vi "09_Notifier_vs_Fronta.vi"() -> ()   [LabVIEW 2019]
panel:
  out "Fronta":dbl(graph)
  out "Notifier":dbl(graph)
  in  "Boolean":bool
  in  "stop":bool
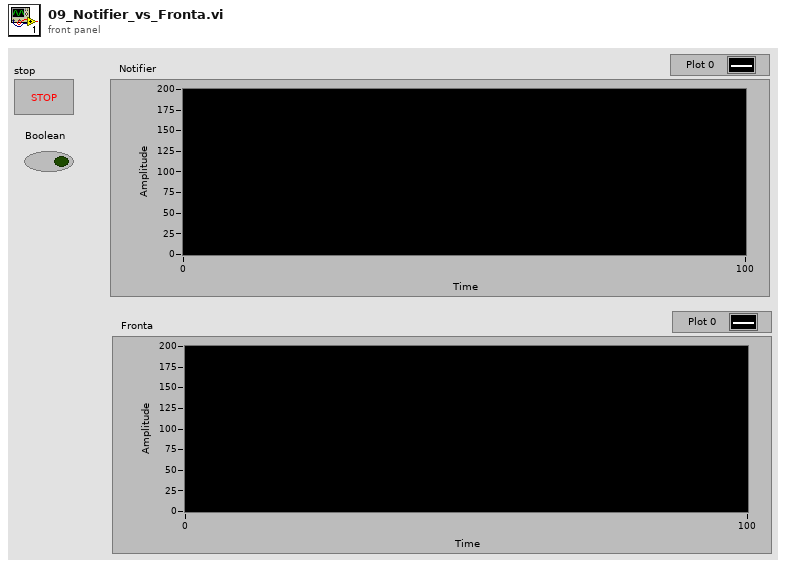
[diagram p1: front panel]
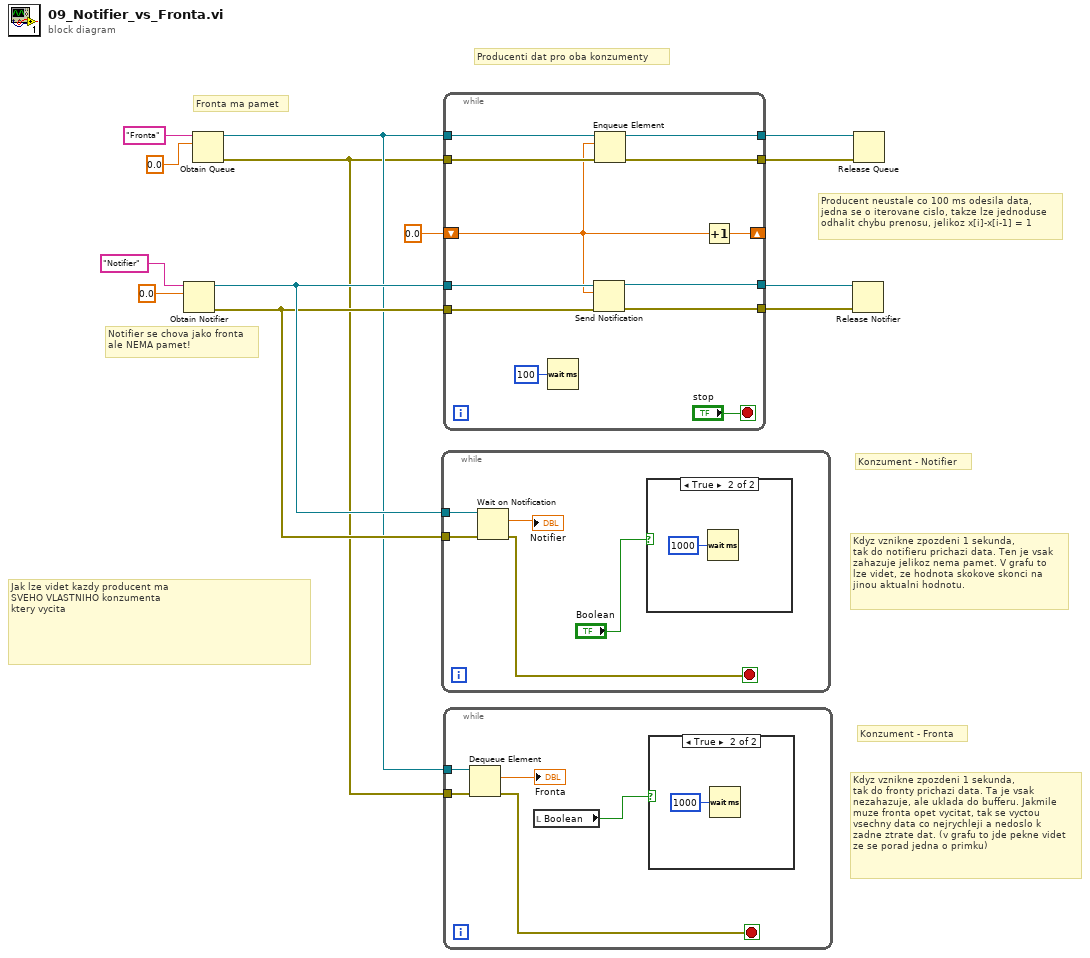
[diagram p0: block diagram]
diagram:
  # "Jak lze videt kazdy producent ma\nSVEHO VLASTNIHO konzumenta\nktery vycita"
  # "Konzument - Fronta"
  # "Konzument - Notifier"
  # "Producenti dat pro oba konzumenty"
  # "Kdyz vznikne zpozdeni 1 sekunda,\ntak do fronty prichazi data. Ta je vsak\nnezahazuje, ale uklada do bufferu. Jakmile\nmuze fronta opet vycitat, tak se vyctou \nvsechny data co nejrychleji a nedoslo k\nzadne ztrate dat. (v grafu to jde pekne videt\nze se porad jedna o primku)"
  # "Producent neustale co 100 ms odesila data,\njedna se o iterovane cislo, takze lze jednoduse\nodhalit chybu prenosu, jelikoz x[i]-x[i-1] = 1"
  # "Kdyz vznikne zpozdeni 1 sekunda,\ntak do notifieru prichazi data. Ten je vsak\nzahazuje jelikoz nema pamet. V grafu to \nlze videt, ze hodnota skokove skonci na \njinou aktualni hodnotu."
  # "Notifier se chova jako fronta\nale NEMA pamet!"
  # "Fronta ma pamet"
  n1 = Obtain Notifier(name (unnamed)="Notifier", notification data type=0.0) -> (notifier out=w8:refnum<notifier>, error out=w7:errorcluster)  [unwired: 2 in, 1 out]
  n2 = Obtain Queue(name (unnamed)="Fronta", element data type=0.0) -> (queue out=w2:refnum<queue>, error out=w1:errorcluster)  [unwired: 3 in, 1 out]
  n3 = while {
    tunnel: w8 -> [w17]
    tunnel: w7 -> [w18]
    stop <- w16 stop-if-true
    n4 = Wait on Notification(notifier=w17, error in (no error)=w18) -> (notification=→"Notifier":dbl, error out=w16:errorcluster)  [unwired: 2 in, 2 out]
    n5 = case shown="True" "Boolean" {
      frame False {
      }
      frame True {
        n6 = Wait (ms)(milliseconds to wait=u32 1000) -> ()  [unwired: 1 out]
      }
    }
  }
  n7 = while {
    tunnel: w8 -> [w31]
    tunnel: w7 -> [w30]
    shift-right: [w28] -> _
    shift-left: 0.0 -> [w20]
    tunnel: [w27] -> w10
    tunnel: [w26] -> w9
    tunnel: w2 -> [w24]
    tunnel: w1 -> [w23]
    tunnel: [w22] -> w4
    tunnel: [w21] -> w3
    stop <- "stop" stop-if-true
    n8 = Wait (ms)(milliseconds to wait=u32 100) -> ()  [unwired: 1 out]
    n9 = Send Notification(notification=w20, notifier=w31, error in (no error)=w30) -> (notifier out=w27:refnum<notifier>, error out=w26:errorcluster)
    n10 = Enqueue Element(queue=w24, element=w20, error in (no error)=w23) -> (queue out=w22:refnum<queue>, error out=w21:errorcluster)  [unwired: 1 in, 1 out]
    n11 = Increment(x=w20) -> (x+1=w28:dbl)
  }
  n12 = while {
    tunnel: w2 -> [w35]
    tunnel: w1 -> [w34]
    stop <- w32 stop-if-true
    n13 = Dequeue Element(queue=w35, error in (no error)=w34) -> (element=→"Fronta":dbl, error out=w32:errorcluster)  [unwired: 1 in, 2 out]
    n14 = local read "Boolean"() -> (w36:bool)
    n15 = case shown="True" w36 {
      frame False {
      }
      frame True {
        n16 = Wait (ms)(milliseconds to wait=u32 1000) -> ()  [unwired: 1 out]
      }
    }
  }
  n17 = Release Notifier(notifier=w10, error in (no error)=w9) -> ()  [unwired: 1 in, 3 out]
  n18 = Release Queue(queue=w4, error in (no error)=w3) -> ()  [unwired: 1 in, 3 out]
